vi "Resetter.vi"(8 "error in":errorcluster) -> (0 "error out 2":errorcluster)   [LabVIEW 2013]
panel:
  in  "stop":bool
  out "Finish Reset":bool
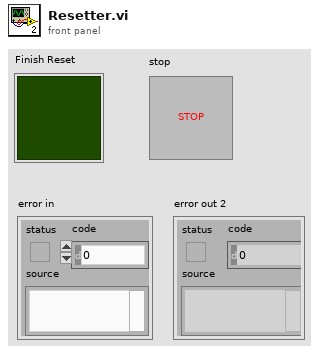
[diagram p1: front panel]
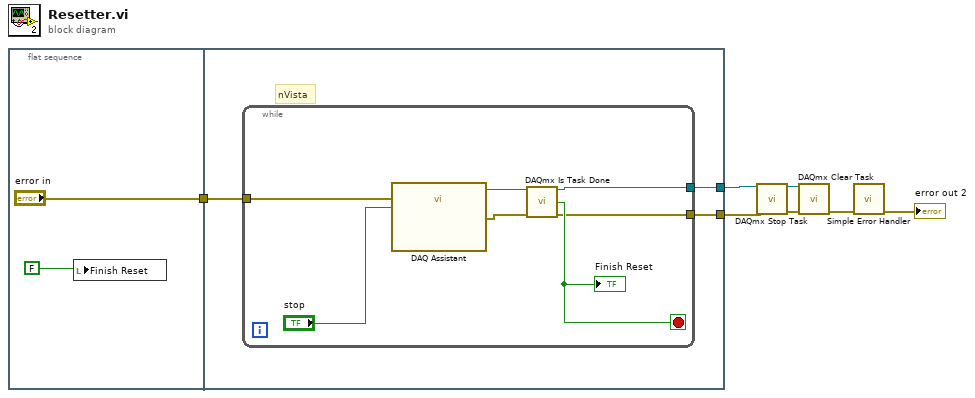
[diagram p0: block diagram]
diagram:
  n1 = flat-sequence {
    tunnel: ["error in"] -> w1
    tunnel: [w12] -> w4
    tunnel: [w11] -> w3
    tunnel: w1 -> [w10]
    frame #0 {
      n2 = local write "Finish Reset"(FALSE) -> ()
    }
    frame #1 {
      # "nVista"
      n3 = while {
        tunnel: [w15] -> w12
        tunnel: [w14] -> w11
        tunnel: w10 -> [w13]
        stop <- w16 stop-if-true
        n4 = call "DAQ Assistant"("error in"=w13, "stop (T)"="stop") -> ("task out"=w18:refnum<k21>, "error out"=w17:errorcluster)  [unwired: 16 in]
        n5 = call <vilib>:"DAQmx Is Task Done.vi"("task/channels in"=w18, "error in"=w17) -> ("task out"=w15:refnum<k21>, "task done?"=w16:bool, "error out"=w14:errorcluster)  [unwired: 11 in]
        "Finish Reset" <- w16
      }
    }
  }
  n6 = call <vilib>:"DAQmx Stop Task.vi"("task/channels in"=w4, "error in"=w3) -> ("task out"=w6:refnum<k21>, "error out"=w7:errorcluster)  [unwired: 12 in]
  n7 = call <vilib>:"DAQmx Clear Task.vi"("task in"=w6, "error in"=w7) -> ("error out"=w5:errorcluster)  [unwired: 13 in]
  n8 = call <vilib>:"Simple Error Handler.vi"("error in (no error)"=w5) -> ("error out"=→"error out 2":errorcluster)  [unwired: 4 in, 4 out]
